vi "Init Flash Cameras.vi"(8 "error in (no error)":errorcluster, 11 "Virtual Camera in":refnum<class "Virtual Camera.lvclass">) -> (0 "error out":errorcluster, 3 "Virtual Camera Out":refnum<class "Virtual Camera.lvclass">)   [LabVIEW 2018, in "Virtual Camera.lvlib" / "Virtual Camera.lvclass"]
uses:
  Virtual Camera.lvclass
  C:/Program Files/National Instruments/LabVIEW 2018/vi.lib/ActorFramework/Actor/Actor.lvclass
  Orca-Flash 4.0 V2/Orca-Flash 4.0 V2.lvclass
  C:/LVCUR/flash-gordon/Hardware/Camera/Camera.lvclass
  Virtual Camera.lvclass/Virtual Camera.ctl
  Resources/GLOBAL/GLOBAL Time-critical.vi
  <vilib>/ActorFramework/Actor/Actor.lvclass
panel:
  out "Array":string[](array[string])
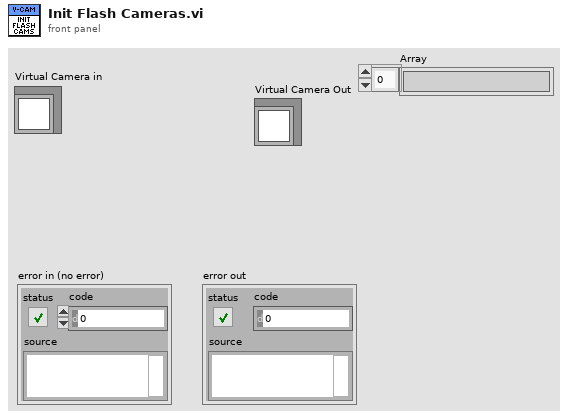
[diagram p1: front panel]
types:
  T1 = typedef "Physical Camera Assignment.ctl" = cluster{"Channel Name":string, "Camera Type":T2, "Serial Number":string, "Flip Vertically":bool, "Flip Horizontally":bool}
  T2 = typedef "Camera Type.ctl" = enum16{"Orca-Flash 4.0 V2"}
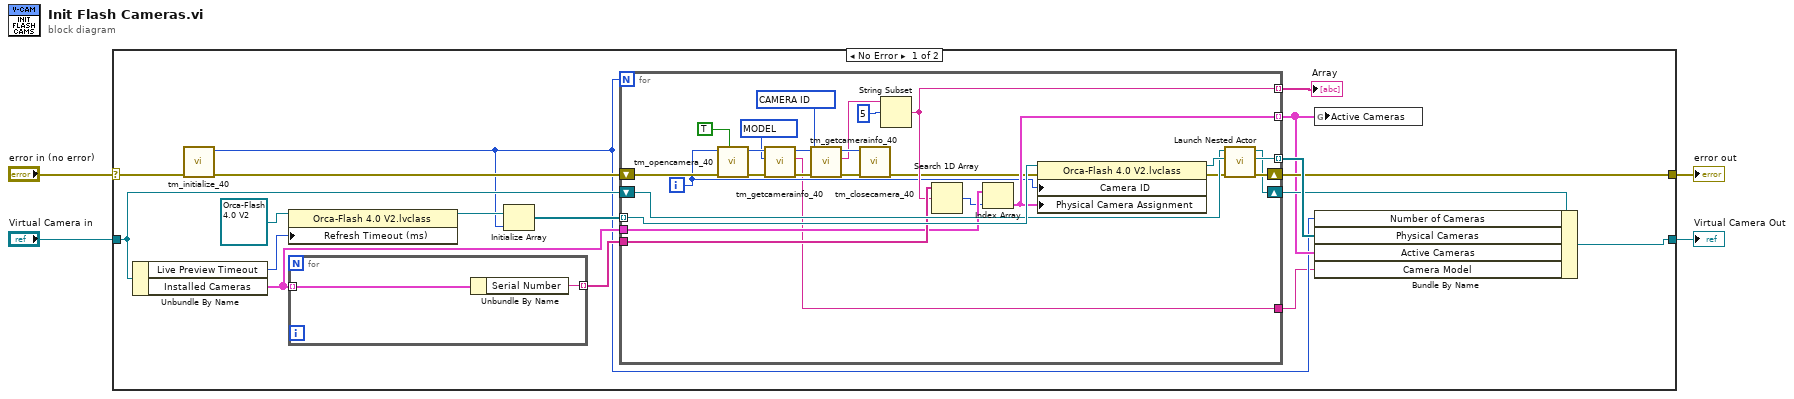
[diagram p0: block diagram]
diagram:
  n1 = case shown="No Error" "error in (no error)" {
    selector: "error in (no error)" -> [w8 w51]
    tunnel: [w18 w51] -> w3
    tunnel: "Virtual Camera in" -> [w16 w52]
    tunnel: [w19 w52] -> w1
    frame No Error {
      n2 = Unbundle By Name(w16) -> ("Live Preview Timeout"=w13:i32, "Installed Cameras"=w11:T1[])
      n3 = call <userlib>:"tm_initialize_40.vi"("error in (no error)"=w8) -> ("error out"=w7:errorcluster, "Number Of Cameras"=w6:u32)  [unwired: 7 in, 2 out]
      n4 = property class="Orca-Flash 4.0 V2.lvclass"(reference=refnum<class "Orca-Flash 4.0 V2.lvclass"> refnum ("Orca-Flash 4.0.lvlib:Orca-Flash 4.0.lvclass"), "Refresh Timeout (ms)"=w13) -> (reference out=w14:refnum<class "Orca-Flash 4.0 V2.lvclass">)  [unwired: 1 in, 1 out]
      n5 = for {
        tunnel: w11 -> [w23] mode=indexing
        tunnel: [w22] -> w12 mode=indexing
        n6 = Unbundle By Name(w23) -> ("Serial Number"=w22:string)
      }
      n7 = Initialize Array(w14, w6) -> (w21:refnum<class "Orca-Flash 4.0 V2.lvclass">[])
      n8 = for {
        N: w6 -> [_]
        tunnel: w21 -> [w48] mode=indexing
        tunnel: [w50] -> w20 mode=indexing
        shift-right: [w49] -> w18
        shift-left: w7 -> [w33]
        shift-right: [w45] -> w17
        shift-left: w16 -> [w46]
        tunnel: w12 -> [w43]
        tunnel: w11 -> [w42]
        tunnel: [w40] -> w9 mode=indexing
        tunnel: [w38] -> w10 mode=indexing
        tunnel: [w24] -> w5
        i -> [w31]
        w25 = u32 67109124 items=["BUS"=67109121, "CAMERA ID"=67109122, "VENDOR"=67109123, "MODEL"=67109124, "CAMERA VERSION"=67109125, "DRIVER VERSION"=67109126, "MODULE VERSIOIN"=67109127, "DCAMAPI VERSION"=67109128] ("Info ID")
        w35 = u32 67109122 items=["BUS"=67109121, "CAMERA ID"=67109122, "VENDOR"=67109123, "MODEL"=67109124, "CAMERA VERSION"=67109125, "DRIVER VERSION"=67109126, "MODULE VERSIOIN"=67109127, "DCAMAPI VERSION"=67109128] ("Info ID")
        n9 = call <userlib>:"tm_opencamera_40.vi"("Force Open"=TRUE, "error in (no error)"=w33, "Camera Index"=w31) -> ("error out"=w26:errorcluster, "Handle out"=w29:u32)  [unwired: 6 in, 1 out]
        n10 = call <userlib>:"tm_getcamerainfo_40.vi"("error in (no error)"=w26, "Info ID"=w25, "Handle in"=w29) -> ("error out"=w27:errorcluster, "String"=w24:string, "Handle out"=w28:u32)  [unwired: 6 in]
        n11 = call <userlib>:"tm_getcamerainfo_40.vi"("error in (no error)"=w27, "Info ID"=w35, "Handle in"=w28) -> ("error out"=w36:errorcluster, "String"=w30:string, "Handle out"=w37:u32)  [unwired: 6 in]
        n12 = call <userlib>:"tm_closecamera_40.vi"("error in (no error)"=w36, "Handle in"=w37) -> ("error out"=w32:errorcluster)  [unwired: 9 in]
        n13 = String Subset(string=w30, offset (0)=5) -> (substring=w38:string)  [unwired: 1 in]
        n14 = Search 1D Array(1D array=w43, element=w38) -> (index of element=w41:i32)  [unwired: 1 in]
        n15 = Index Array(array=w42, index=w41) -> (element=w40:T1)
        n16 = property class="Orca-Flash 4.0 V2.lvclass"(reference=w48, error in=w32, "Camera ID"=w31, "Physical Camera Assignment"=w40) -> (reference out=w47:refnum<class "Orca-Flash 4.0 V2.lvclass">, error out=w44:errorcluster)
        n17 = call <vilib>:"Launch Nested Actor.vi"("error in (no error)"=w44, "Nested Actor"=w47, "Caller Actor in"=w46) -> ("error out"=w49:errorcluster, "Nested Actor's Enqueuer"=w50:refnum<class "Message Enqueuer.lvclass">, "Caller Actor out"=w45:refnum<class "Virtual Camera.lvclass">)  [unwired: 6 in]
      }
      "Array" <- w10
      n18 = global write "GLOBAL Time-critical.vi" "Active Cameras"(w9) -> ()
      n19 = Bundle By Name(cluster=w17, "Number of Cameras"=w6, "Physical Cameras"=w20, "Active Cameras"=w9, "Camera Model"=w5) -> (w19:refnum<class "Virtual Camera.lvclass">)
    }
    frame Error {
    }
  }
  "error out" <- w3
  "Virtual Camera Out" <- w1
